vi "FormatMeas.vi"(0 "VISA IN":refnum<visa-resource-name>, 4 "Format":string(combo)="MLINear", 5 "error in":errorcluster, 7 "Channel":i32=1) -> (14 "VISA Out":refnum<visa-resource-name>, 19 "error out":errorcluster)   [LabVIEW 2018, in "PNA-X.lvlib"]
doc: "CALCulate<cnum>:FORMat <char> \n(Read-Write) Sets the display format for the measurement. \nSee Critical Note \nParameters \n<cnum> Channel number of the measurement. There must be a selected measurement \non that channel. If unspecified, <cnum> is set to 1. \n<char> Choose from: \nMLINear \nMLOGarithmic \nPHASe \nUPHase 'Unwrapped phase \nIMAGinary \nREAL \nPOLar \nSMITh \nSADMittance 'Smith Admittance \nSWR \nGDELay 'Group Delay \n1512\n\nExamples CALC:FORM MLIN \ncalculate2:format polar \nQuery Syntax CALCulate<cnum>:FORMat? \nReturn Type Character \nDefault MLINear \n1513\n\nCalculate:FSimulator Commands \nSpecifies settings and fixturing for Balanced Measurements. \nClick a blue keyword to view the command details. \nSee Also \nExample Programs \nSCPI Command Tree"
uses:
  PNA-X.lvlib
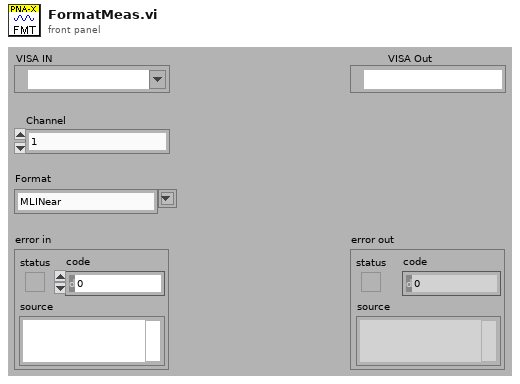
[diagram p1: front panel]
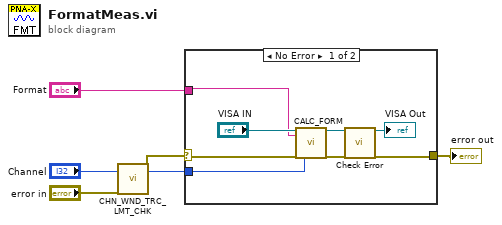
[diagram p0: block diagram]
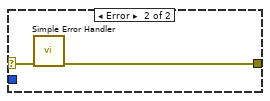
[diagram p2: hidden frame]
diagram:
  n1 = call "CHN_WND_TRC_LMT_CHK.vi"("Channel"="Channel", "error in"="error in") -> ("error out"=w1:errorcluster, "Channel"=w4:i32)  [unwired: 13 in, 3 out]
  n2 = case shown="No Error" w1 {
    selector: w1 -> [w12 w16]
    tunnel: [w14 w15] -> w5
    tunnel: w4 -> [w10 _]
    tunnel: "Format" -> [w9 _]
    frame No Error {
      n3 = call "CALC_FORM.vi"("VISA IN"="VISA IN", "Format"=w9, "error in"=w12, "Channel"=w10) -> ("VISA Out"=w8:refnum<visa-resource-name>, "error out"=w7:errorcluster)  [unwired: 14 in]
      n4 = call "Check Error.vi"("VISA Resource Name"=w8, "error in (no error)"=w7) -> ("dup VISA session"=→"VISA Out":refnum<visa-resource-name>, "error out"=w14:errorcluster)  [unwired: 16 in]
    }
    frame Error {
      n5 = call <vilib>:"Simple Error Handler.vi"("error in (no error)"=w16) -> ("error out"=w15:errorcluster)  [unwired: 4 in, 4 out]
    }
  }
  "error out" <- w5
